vi "MensajesAlarmas.vi"() -> ()   [LabVIEW 2018]
panel:
  in  "Modulación de Voltaje V3_V1 en Generador 1 sobrepasada":string
  in  "Modulación de Voltaje V2_V3 en Generador 1 sobrepasada":string
  in  "Modulación de Voltaje V1_V2 en Generador 1 sobrepasada":string
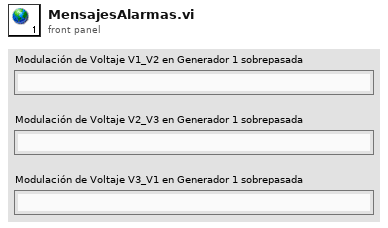
[diagram p1: front panel]
diagram:
